vi "lab2_question4.vi"() -> ()   [LabVIEW 2019]
uses:
  <vilib>/Platform/TimedLoop/XDataNode/timing_clust.ctl
  <vilib>/Platform/TimedLoop/XDataNode/nitl_modes.ctl
  <vilib>/Platform/TimedLoop/XDataNode/wakeup.ctl
  <vilib>/Analysis/3filter.llb/Filter Passband Type.ctl
  <vilib>/DAQmx/read.llb/DAQmx Read (Analog DBL 1Chan 1Samp).vi
  <vilib>/DAQmx/create/channels.llb/DAQmx Create Channel (AI-Voltage-Basic).vi
  <vilib>/DAQmx/miscellaneous.llb/DAQmx Fill In Error Info.vi
  <vilib>/platform/TimedLoop/XDataNode/XDataNode.xnode
  <vilib>/Platform/TimedLoop/XDataNode/XDNodeRunTimeDep.lvlib
  <vilib>/Analysis/NI_AALBase.lvlib
  <vilib>/ptbypt/NI_PtbyPt.lvlib
panel:
  out "Iteration":i32
  out "Raw Position":dbl
  out "Raw Position Graph":dbl(graph)
  out "Raw Acceleration":dbl
  out "Raw Velocity":dbl
  out "Filtered Velocity":dbl
  out "Filtered Velocity Graph":dbl(graph)
  in  "low cutoff freq:  Velocity":dbl=0.125 format="%0.3f"
  out "Filtered Acceleration":dbl
  out "Filtered Acceleration Graph":dbl(graph)
  in  "low cutoff freq: Acceleration":dbl=0.125 format="%0.3f"
  out "Raw Acceleration Graph":dbl(graph)
  out "Raw Veloctiy Graph":dbl(graph)
  in  "low cutoff freq: Position":dbl=0.125 format="%0.3f"
  out "Filtered Postion Graph":dbl(graph)
  out "Filtered Position":dbl
  in  "STOP":bool
  out "Position":dbl(knob) scale=-32.5..32.5
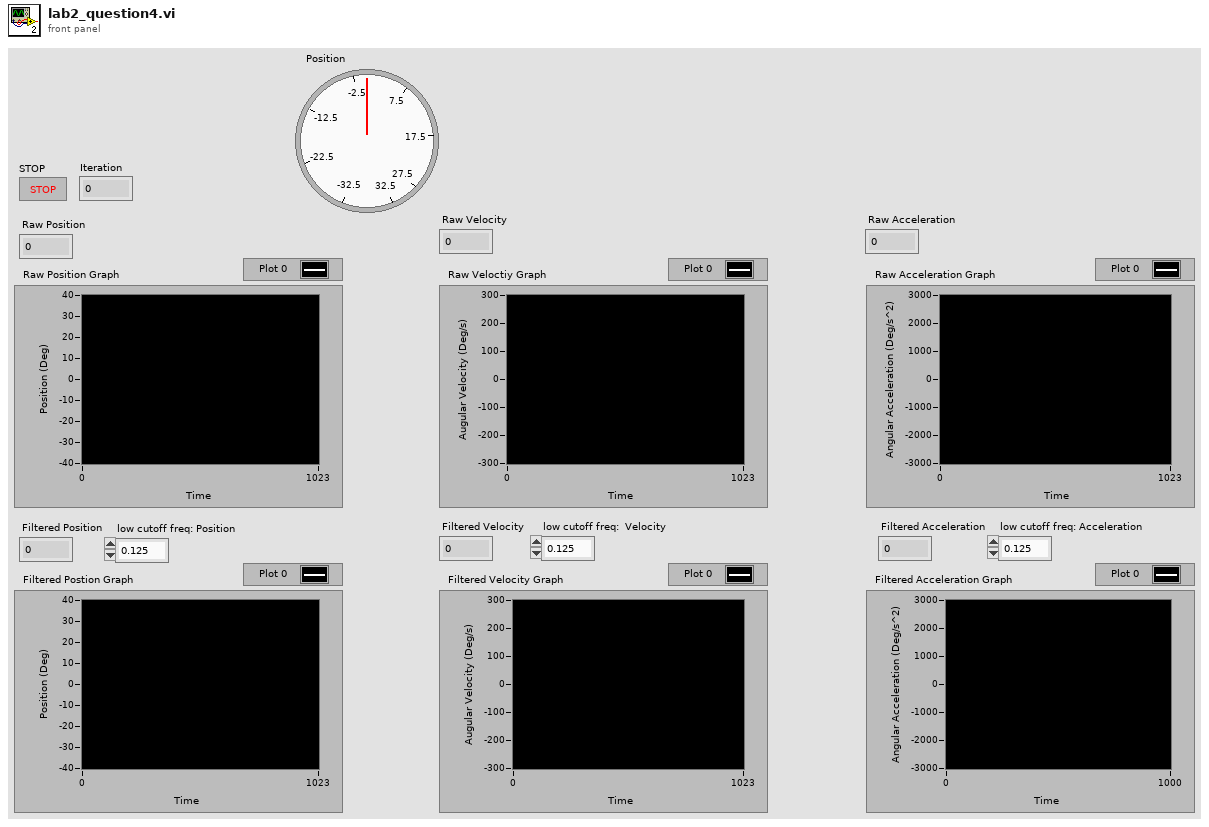
[diagram p1: front panel]
types:
  T1 = typedef "NI_AALBase.lvlib/Filter Passband Type.ctl" = enum32{"Lowpass", "Highpass", "Bandpass", "Bandstop"}
  T2 = typedef "XDNodeRunTimeDep.lvlib/timing_clust.ctl" = cluster{"Expected End [f-1]":u64, "Actual End [f-1]":u64, "Finished Late? [f-1]":bool, "Expected End [i-1]":u64, "Actual End [i-1]":u64, "Finished Late? [i-1]":bool, "Expected Start [i]":u64, "Actual Start [i]":u64, "Expected Start [f]":u64, "Actual Start [f]":u64, "Source Name":string, "Structure Name":string, "Period":i64, "Deadline":i64, "Offset":i64, "Start":i64, "Priority":i32, "Timeout":i32, "Mode":T3, "Wakeup Reason":T4, "Error":errorcluster, "Source Type":string, "Secondary Source Type":string, "Global End Time":u64, "Global Start Time":u64, "Frame Duration":u64, "Iteration Duration":u64, "Assigned CPU":i32, "I/O Scan Engine Mode":u32}
  T3 = typedef "XDNodeRunTimeDep.lvlib/nitl_modes.ctl" = enum32{"No Change", "Process missed periods, maintain original phase", "Discard missed periods, maintain original phase", "Process missed periods, ignore original phase", "Discard missed periods, ignore original phase"}
  T4 = typedef "XDNodeRunTimeDep.lvlib/wakeup.ctl" = enum32{"Normal", "Aborted", "Asynchronous wakeup", "Timing source error", "Timed loop error", "Timeout"}
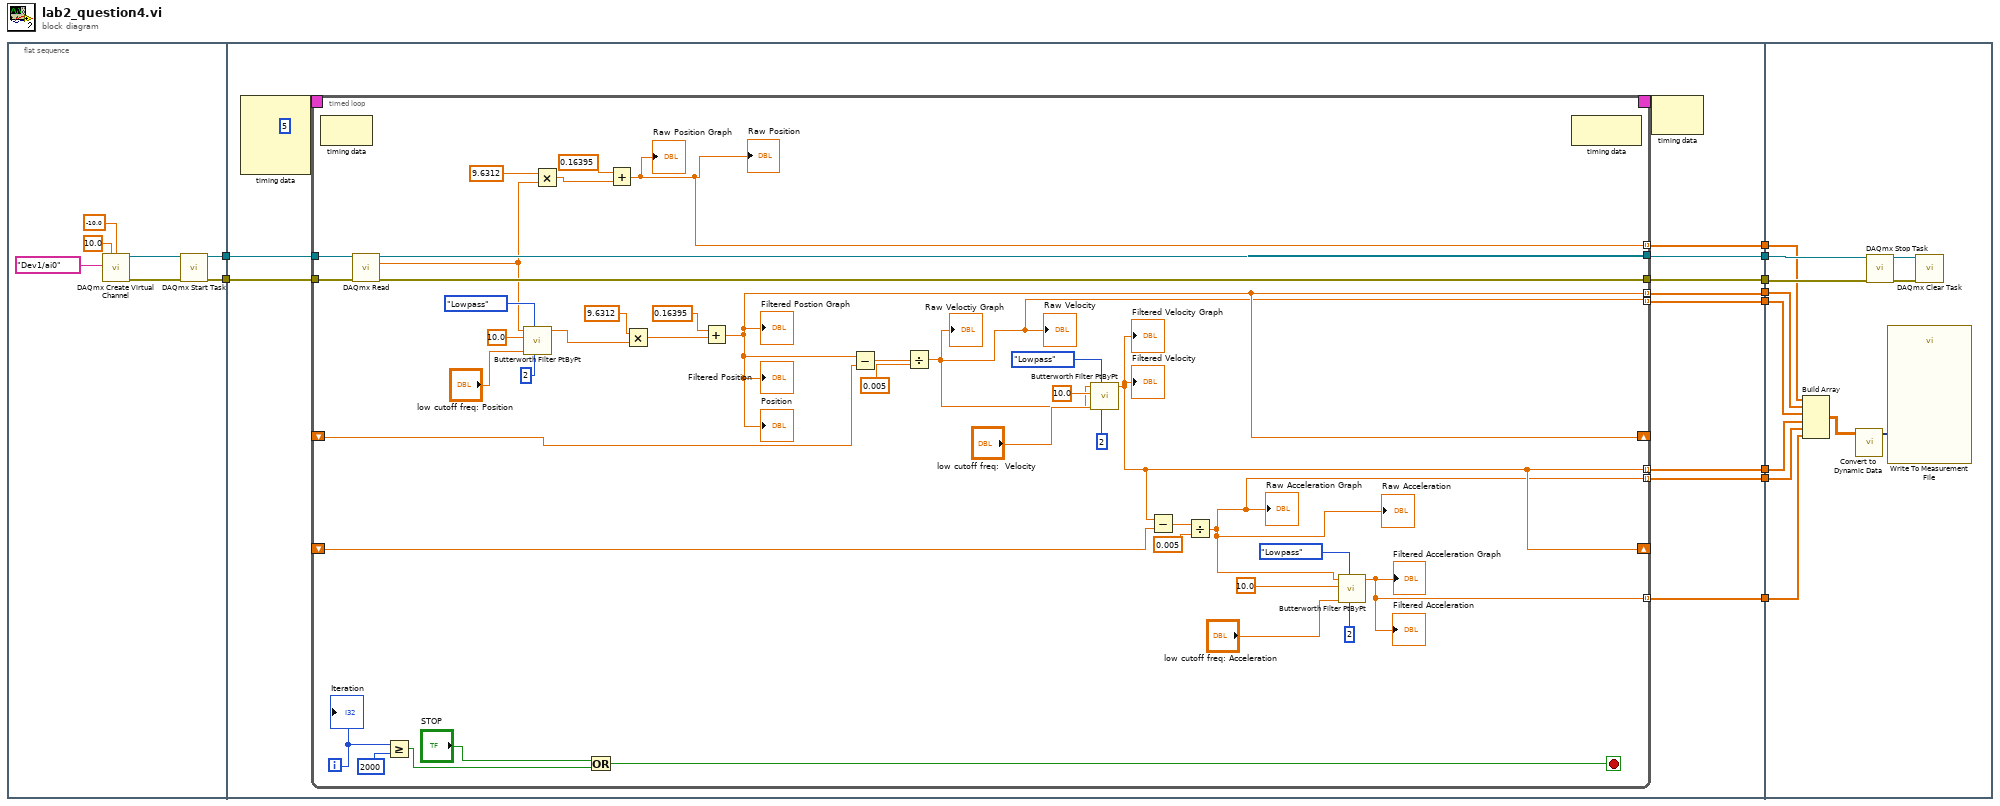
[diagram p0: block diagram]
diagram:
  n1 = flat-sequence {
    tunnel: [w13] -> w10
    tunnel: [w11] -> w9
    tunnel: w10 -> [w28]
    tunnel: [w27] -> w8
    tunnel: w9 -> [w26]
    tunnel: [w24] -> w7
    tunnel: [w23] -> w6
    tunnel: [w22] -> w5
    tunnel: [w21] -> w4
    tunnel: [w20] -> w3
    tunnel: [w19] -> w2
    tunnel: [w18] -> w1
    tunnel: w8 -> [w89]
    tunnel: w7 -> [w87]
    tunnel: w6 -> [w83]
    tunnel: w5 -> [w81]
    tunnel: w4 -> [w79]
    tunnel: w3 -> [w84]
    tunnel: w2 -> [w82]
    tunnel: w1 -> [w80]
    frame #0 {
      n2 = call-poly <vilib>:"DAQmx Create Virtual Channel.vi"("maximum value"=10.0, "minimum value"=-10.0, "physical channels"=tag "Dev1/ai0") -> ("task out"=w12:refnum<k21>, "error out"=w14:errorcluster)  [unwired: 11 in]
      n3 = call <vilib>:"DAQmx Start Task.vi"("task/channels in"=w12, "error in"=w14) -> ("task out"=w11:refnum<k21>, "error out"=w13:errorcluster)  [unwired: 12 in]
    }
    frame #1 {
      n4 = node-c288(i64 5 ("Period")) -> (w30:T2)  [unwired: 3 in]
      n5 = timed-loop {
        timing: w30 -> [_]
        timing-out: [_] -> w29
        tunnel: w28 -> [w71]
        tunnel: [w70] -> w27
        tunnel: w26 -> [w65]
        tunnel: [w64] -> w24
        shift-right: [w36] -> _
        shift-left: _ -> [w42]
        shift-right: [w35] -> _
        shift-left: _ -> [w61]
        tunnel: [w36] -> w23 mode=indexing
        tunnel: [w35] -> w22 mode=indexing
        tunnel: [w34] -> w21 mode=indexing
        tunnel: [w33] -> w20 mode=indexing
        tunnel: [w32] -> w19 mode=indexing
        tunnel: [w31] -> w18 mode=indexing
        i -> [w40]
        stop <- w37 stop-if-true
        n6 = node-c288() -> ()  [unwired: 1 in, 1 out]
        n7 = call-poly <vilib>:"DAQmx Read.vi"("task/channels in"=w65, "error in"=w71) -> ("task out"=w64:refnum<k21>, "data"=w47:dbl, "error out"=w70:errorcluster)  [unwired: 11 in]
        n8 = Greater Or Equal?(x=w40, y=2000) -> (x >= y?=w41:bool)
        n9 = call <vilib>:"Butterworth Filter PtByPt.vi"("order"=2, "filter type"=Filter_Passband_Type."Lowpass", "low cutoff freq: fl"="low cutoff freq: Position", "sampling freq: fs"=10.0, "x"=w47) -> ("Filtered x"=w43:dbl)  [unwired: 4 in, 1 out]
        n10 = Multiply(x=9.6312, y=w47) -> (x*y=w49:dbl)
        n11 = Or(x="STOP", y=w41) -> (x .or. y?=w37:bool)
        n12 = Add(x=0.16395, y=w49) -> (x+y=w33:dbl)
        "Raw Position Graph" <- w33
        "Raw Position" <- w33
        n13 = Multiply(x=9.6312, y=w43) -> (x*y=w45:dbl)
        n14 = Add(x=0.16395, y=w45) -> (x+y=w36:dbl)
        "Filtered Postion Graph" <- w36
        "Filtered Position" <- w36
        "Position" <- w36
        n15 = Subtract(x=w36, y=w42) -> (x-y=w63:dbl)
        n16 = Divide(x=w63, y=0.005) -> (x/y=w32:dbl)
        "Raw Veloctiy Graph" <- w32
        "Raw Velocity" <- w32
        n17 = call <vilib>:"Butterworth Filter PtByPt.vi"("order"=2, "filter type"=Filter_Passband_Type."Lowpass", "low cutoff freq: fl"="low cutoff freq:  Velocity", "sampling freq: fs"=10.0, "x"=w32) -> ("Filtered x"=w35:dbl)  [unwired: 4 in, 1 out]
        "Filtered Velocity Graph" <- w35
        "Filtered Velocity" <- w35
        n18 = Subtract(x=w35, y=w61) -> (x-y=w60:dbl)
        n19 = Divide(x=w60, y=0.005) -> (x/y=w31:dbl)
        "Raw Acceleration Graph" <- w31
        "Raw Acceleration" <- w31
        n20 = call <vilib>:"Butterworth Filter PtByPt.vi"("order"=2, "filter type"=Filter_Passband_Type."Lowpass", "low cutoff freq: fl"="low cutoff freq: Acceleration", "sampling freq: fs"=10.0, "x"=w31) -> ("Filtered x"=w34:dbl)  [unwired: 4 in, 1 out]
        "Filtered Acceleration Graph" <- w34
        "Filtered Acceleration" <- w34
        n21 = node-c288() -> ()  [unwired: 1 in, 1 out]
        "Iteration" <- w40
      }
      n22 = node-c288(w29) -> ()  [unwired: 1 out]
    }
    frame #2 {
      n23 = Build Array(w84, w83, w82, w81, w80, w79) -> (w78:dbl[][])
      n24 = call "Convert to Dynamic Data"("2D Array"=w78) -> ("Dynamic Data Type"=w85:dynamicdata)  [unwired: 3 in]
      n25 = call <vilib>:"DAQmx Stop Task.vi"("task/channels in"=w87, "error in"=w89) -> ("task out"=w86:refnum<k21>, "error out"=w88:errorcluster)  [unwired: 12 in]
      n26 = call "Write To Measurement File"("Signals"=w85) -> ()  [unwired: 16 in, 3 out]
      n27 = call <vilib>:"DAQmx Clear Task.vi"("task in"=w86, "error in"=w88) -> ()  [unwired: 13 in, 1 out]
    }
  }
